vi "Arm Setup.vi"() -> ()   [LabVIEW 2018]
uses:
  <vilib>/robotics/Kinematics/DH Kinematic Parameters.ctl
  <vilib>/robotics/Kinematics/Link/Joint Type.ctl
  <vilib>/robotics/Kinematics/Analytical/Initialize Generic Serial Arm.vi
  <vilib>/picture/3D Picture Control/Object/Add Object (reference).vi
  <vilib>/robotics/Kinematics/Analytical/NI_Robotics_AnalyticKinematics.lvlib
  <vilib>/robotics/Kinematics/Plotting/NI_Robotics_3DKinematics.lvlib
  <vilib>/picture/3D Picture Control/NI_3D Picture Control.lvlib
  <vilib>/robotics/Kinematics/NI_Kinematics.lvlib
  <vilib>/robotics/Kinematics/Robot/NI_Robotics_Serial Robot Arm.lvclass
  <vilib>/robotics/Kinematics/Link/NI_Robotics_Link.lvclass
panel:
  in  "joint positions":dbl[](array[numeric])
  in  "Start Z":dbl
  in  "Start Y":dbl
  in  "Start X":dbl
  in  "End Y":dbl
  in  "End Z":dbl
  in  "End X":dbl
  out "3D Picture Control":refnum<vi>(3d-picture)
  in  "kinematic parameters":T1[](array[typedef])=[{"twist angle"=0.0, "length"=220.0, "rotation angle"=0.0, "offset distance"=20.85, "joint type"=enum."Revolute", "joint coordinate offset"=0.0}, {"twist angle"=0.0, "length"=200.0, "rotation angle"=0.0, "offset distance"=20.85, "joint type"=enum."Revolute", "joint coordinate offset"=0.0}, {"twist angle"=0.0, "length"=180.0, "rotation angle"=0.0, "offset distance"=20.85, "joint type"=enum."Revolute", "joint coordinate offset"=0.0}, {"twist angle"=0.0, "length"=0.0, "rotation angle"=0.0, "offset distance"=0.0, "joint type"=enum."Revolute", "joint coordinate offset"=0.0}]
  in  "error in (no error)":errorcluster
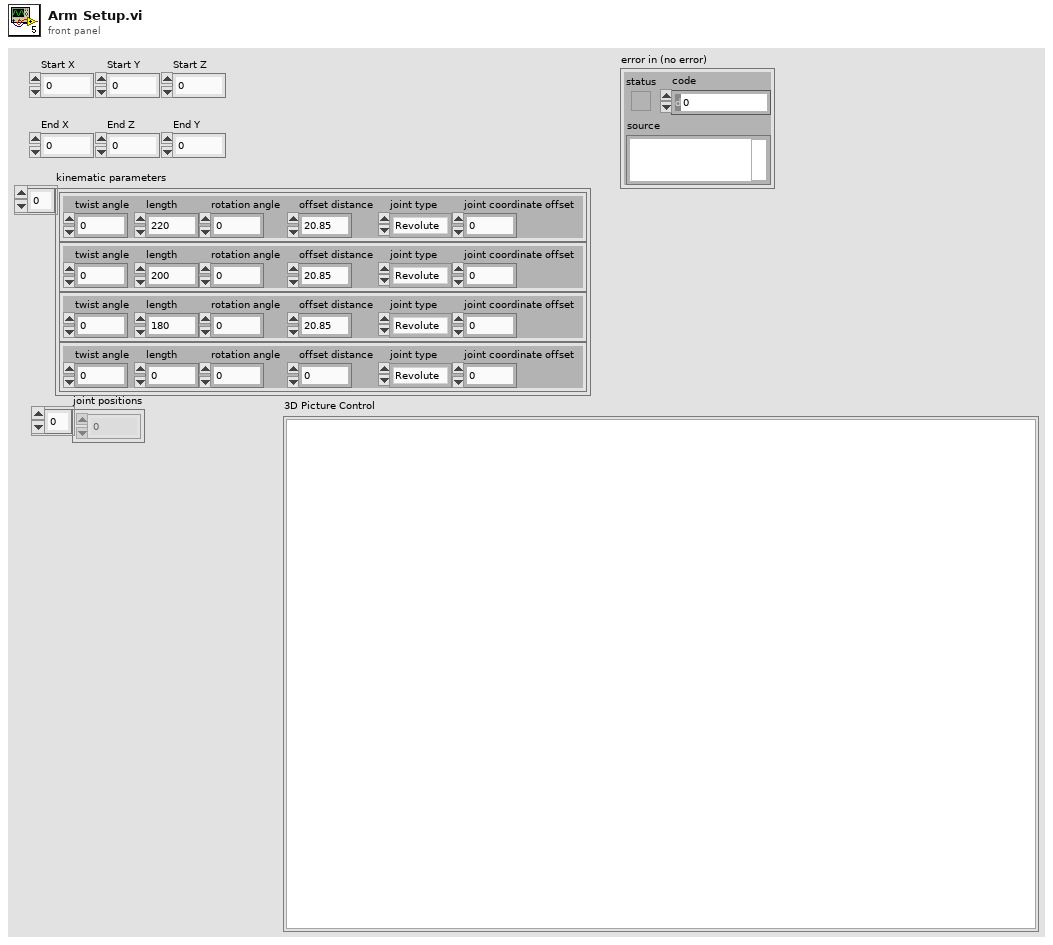
[diagram p1: front panel]
types:
  T1 = typedef "DH Kinematic Parameters.ctl" = cluster{"twist angle":dbl, "length":dbl, "rotation angle":dbl, "offset distance":dbl, "joint type":T2, "joint coordinate offset":dbl}
  T2 = typedef "NI_Robotics_Link.lvclass/Joint Type.ctl" = enum16{"Revolute", "Prismatic"}
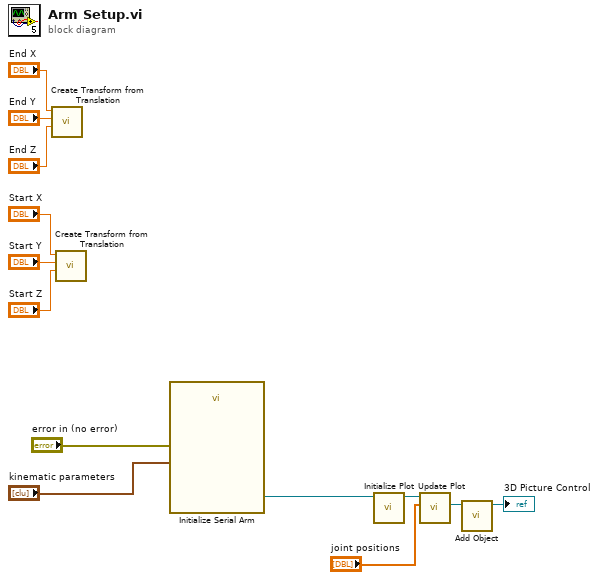
[diagram p0: block diagram]
diagram:
  n1 = call <vilib>:"Create Transform from Translation.vi"("z"="End Z", "y"="End Y", "x"="End X") -> ()  [unwired: 8 in, 1 out]
  n2 = call <vilib>:"Create Transform from Translation.vi"("z"="Start Z", "y"="Start Y", "x"="Start X") -> ()  [unwired: 8 in, 1 out]
  n3 = call-poly <vilib>:"Initialize Serial Arm.vi"("error in (no error)"="error in (no error)", "kinematic parameters"="kinematic parameters") -> ("serial arm out"=w3:refnum<class "NI_Robotics_Serial Robot Arm.lvclass">)  [unwired: 8 in, 1 out]
  n4 = call <vilib>:"Initialize Plot.vi"("serial arm in"=w3) -> ("serial arm out"=w10:refnum<class "NI_Robotics_Serial Robot Arm.lvclass">)  [unwired: 9 in, 1 out]
  n5 = call <vilib>:"Update Plot.vi"("joint positions"="joint positions", "serial arm in"=w10) -> ("serial arm scene"=w1:refnum<vi>)  [unwired: 7 in, 2 out]
  n6 = call-poly <vilib>:"Add Object.vi"("Scene Object In"=w1) -> ("Scene Object Out"=→"3D Picture Control":refnum<vi>)  [unwired: 8 in, 2 out]
